vi "rozgrywka (subvi).vi"(8 "Array":dbl[][](array[numeric]), 9 "wiersz":i32, 10 "kolumna":i32, 11 "VKey":T1) -> (0 "Po ogonie":bool, 1 "przegrana?":bool=TRUE, 2 "Array 2":dbl[][](array[numeric]), 3 "zjadł?":bool)   [LabVIEW 2020]
uses:
  <vilib>/event_ctls.llb/eventvkey.ctl
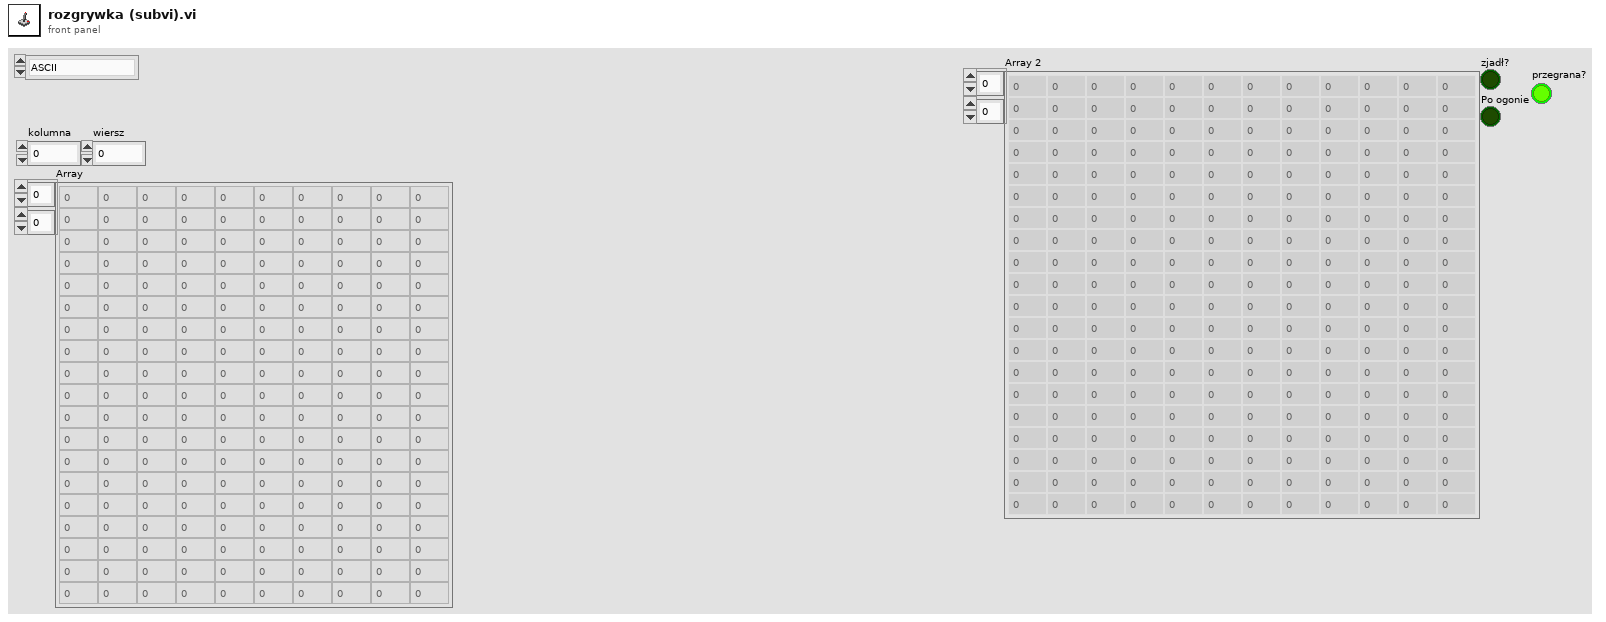
[diagram p1: front panel]
types:
  T1 = typedef "eventvkey.ctl" = enum16{"ASCII", "Enter", "Return", "Shift", "Ctrl", "Alt", "Cmd", "Opt", "Caps", "NumLock", "Clear", "Break", "Up", "Down", "Left", "Right", "Insert", "Delete", "Home", "End", "PageUp", "PageDown", "Escape", "Help", "Pause", "ScrollLock", "F1", "F2", "F3", "F4", "F5", "F6", "F7", "F8", "F9", "F10", "F11", "F12", "F13", "F14", "F15", "F16", "F17", "F18", "F19", "F20", "F21", "F22", "F23", "F24", "Play", "VolumeUp", "VolumeDown", "Mute", "Two Byte Char"}
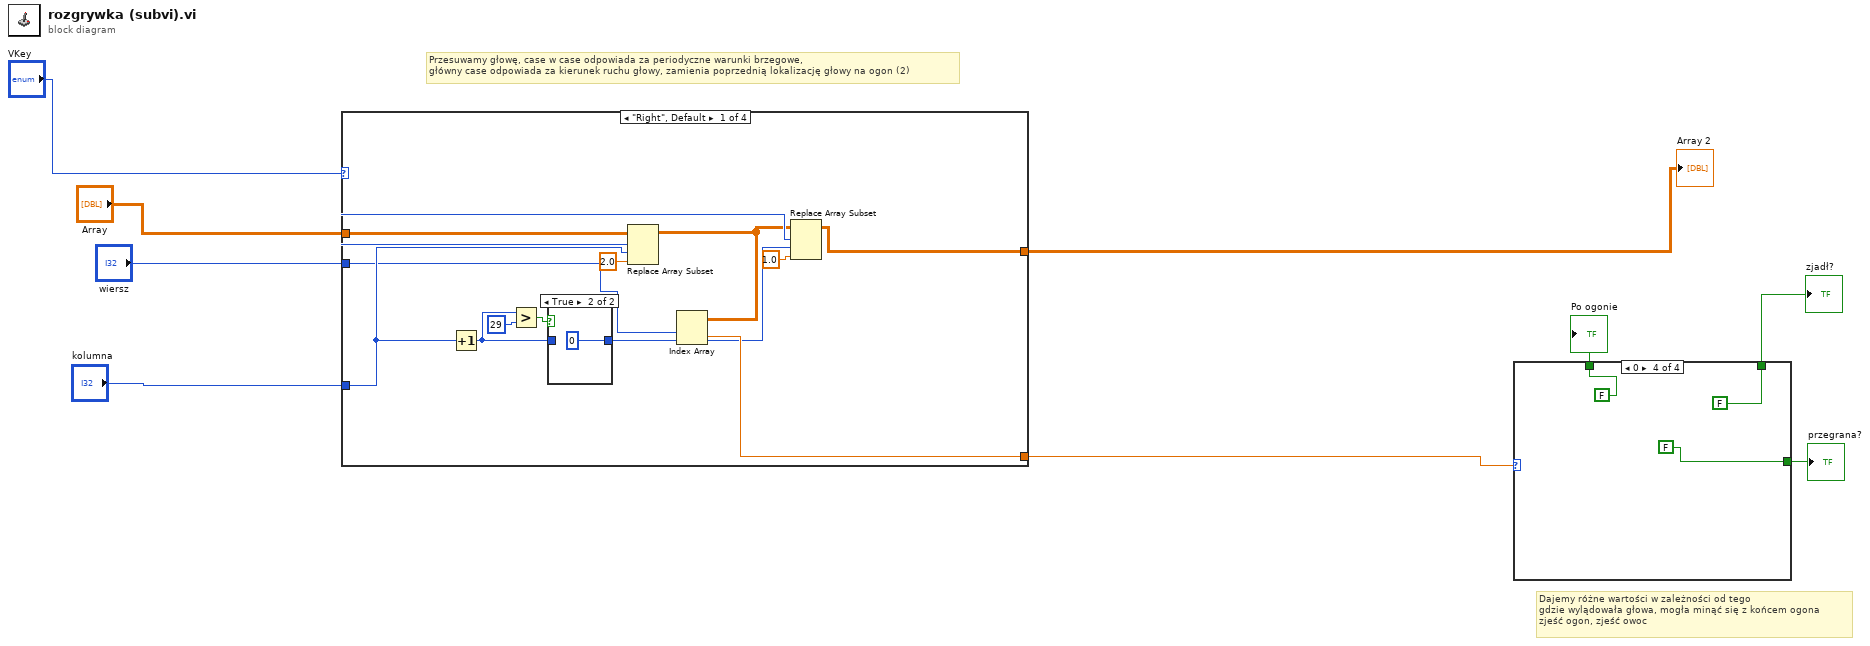
[diagram p0: block diagram]
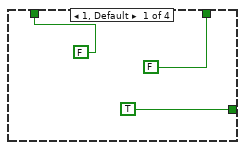
[diagram p2: hidden frame]
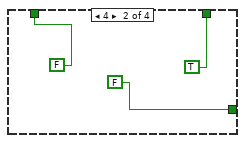
[diagram p3: hidden frame]
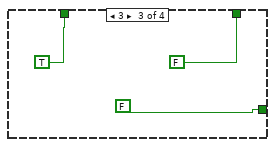
[diagram p4: hidden frame]
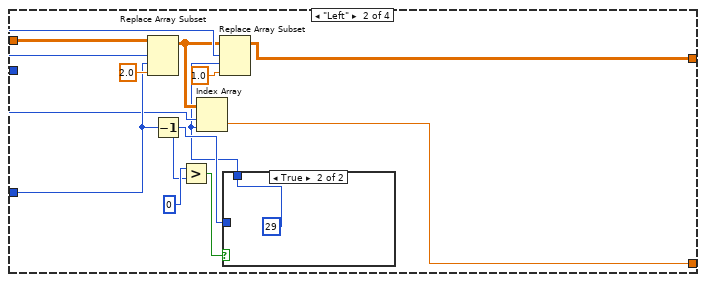
[diagram p6: hidden frame]
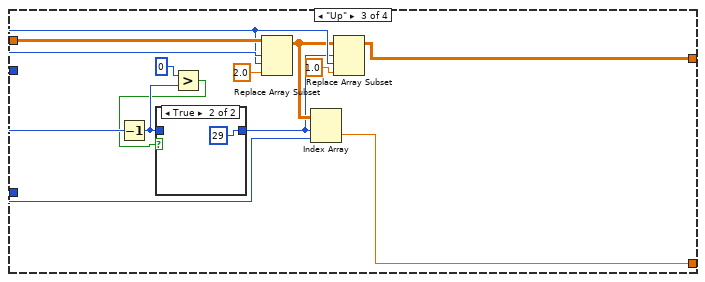
[diagram p8: hidden frame]
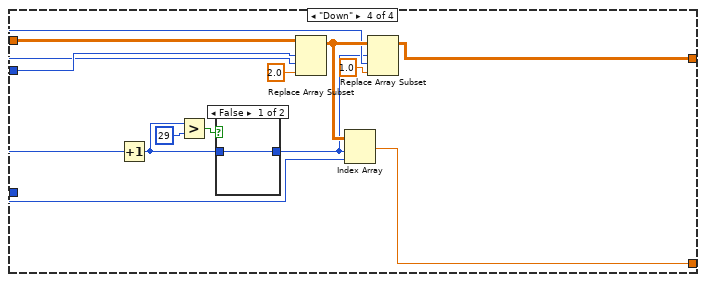
[diagram p10: hidden frame]
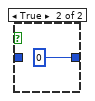
[diagram p11: hidden frame]
diagram:
  # "Przesuwamy głowę, case w case odpowiada za periodyczne warunki brzegowe,\ngłówny case odpowiada za kierunek ruchu głowy, zamienia poprzednią lokalizację głowy na ogon (2)"
  # "Dajemy różne wartości w zależności od tego\ngdzie wylądowała głowa, mogła minąć się z końcem ogona\nzjeść ogon, zjeść owoc"
  n1 = case shown="\"Right\", Default" "VKey" {
    tunnel: [w19 w33 w47 w61] -> w9
    tunnel: "Array" -> [w21 w35 w49 w63]
    tunnel: "kolumna" -> [w17 w31 w44 w57]
    tunnel: "wiersz" -> [w16 w30 w45 w59]
    tunnel: [w14 w28 w42 w56] -> w4
    frame "Right", Default {
      n2 = Increment(x=w17) -> (x+1=w13:i32)
      n3 = Greater?(x=w13, y=29) -> (0:w10:bool)
      n4 = case shown="True" w10 {
        tunnel: w13 -> [w22 _]
        tunnel: [w22 0] -> w12
        frame False {
        }
        frame True {
        }
      }
      n5 = Replace Array Subset(array=w21, new element=2.0 ("new element/subarray"), index (row)=w16, index (col)=w17) -> (w15:dbl[][])
      n6 = Index Array(array=w15, index (row)=w16, index (col)=w12) -> (element=w14:dbl)
      n7 = Replace Array Subset(array=w15, new element=1.0 ("new element/subarray"), index (row)=w16, index (col)=w12) -> (w19:dbl[][])
    }
    frame "Left" {
      n8 = Replace Array Subset(array=w35, new element=2.0 ("new element/subarray"), index (row)=w30, index (col)=w31) -> (w29:dbl[][])
      n9 = Decrement(x=w31) -> (x-1=w26:i32)
      n10 = Greater?(x=0 ("y"), y=w26) -> (0:w24:bool)
      n11 = case shown="True" w24 {
        tunnel: w26 -> [w36 _]
        tunnel: [w36 29] -> w25
        frame False {
        }
        frame True {
        }
      }
      n12 = Index Array(array=w29, index (row)=w30, index (col)=w25) -> (element=w28:dbl)
      n13 = Replace Array Subset(array=w29, new element=1.0 ("new element/subarray"), index (row)=w30, index (col)=w25) -> (w33:dbl[][])
    }
    frame "Up" {
      n14 = Decrement(x=w45) -> (x-1=w40:i32)
      n15 = Greater?(x=0 ("y"), y=w40) -> (0:w38:bool)
      n16 = case shown="True" w38 {
        tunnel: w40 -> [w50 _]
        tunnel: [w50 29] -> w39
        frame False {
        }
        frame True {
        }
      }
      n17 = Replace Array Subset(array=w49, new element=2.0 ("new element/subarray"), index (row)=w45, index (col)=w44) -> (w43:dbl[][])
      n18 = Index Array(array=w43, index (row)=w39, index (col)=w44) -> (element=w42:dbl)
      n19 = Replace Array Subset(array=w43, new element=1.0 ("new element/subarray"), index (row)=w39, index (col)=w44) -> (w47:dbl[][])
    }
    frame "Down" {
      n20 = Increment(x=w59) -> (x+1=w53:i32)
      n21 = Greater?(x=w53, y=29) -> (0:w54:bool)
      n22 = case shown="False" w54 {
        tunnel: w53 -> [w64 _]
        tunnel: [w64 0] -> w52
        frame False {
        }
        frame True {
        }
      }
      n23 = Replace Array Subset(array=w63, new element=2.0 ("new element/subarray"), index (row)=w59, index (col)=w57) -> (w58:dbl[][])
      n24 = Index Array(array=w58, index (row)=w52, index (col)=w57) -> (element=w56:dbl)
      n25 = Replace Array Subset(array=w58, new element=1.0 ("new element/subarray"), index (row)=w52, index (col)=w57) -> (w61:dbl[][])
    }
  }
  "Array 2" <- w9
  n26 = case shown="0" w4 {
    tunnel: [TRUE FALSE FALSE FALSE] -> w3
    tunnel: [FALSE TRUE FALSE FALSE] -> w2
    tunnel: [FALSE FALSE TRUE FALSE] -> w1
    frame 1, Default {
    }
    frame 4 {
    }
    frame 3 {
    }
    frame 0 {
    }
  }
  "zjadł?" <- w2
  "przegrana?" <- w3
  "Po ogonie" <- w1
